vi "S4GUI.vi"(7 "Tab ObsEng":enum32{"Obs", "CCD modes", "Guider", "Eng"}(tab)) -> ()   [LabVIEW 2018] (continued)
        n1953 = event-data() -> ()  [unwired: 1 in, 6 out]
        n1954 = disable-structure shown="Disabled" {
          disable-tunnel: w3779 -> [w3791 _]
          frame Disabled {
            # "como alterar o valor de um parametro em \"Parameter Input\""
            n1955 = Unbundle By Name(w3791) -> ("Parameters"=w3793:T5)
            n1956 = Bundle By Name(cluster=w3793, "Readout\nRate"=u8 1 ("Readout\nRate")) -> (w3790:T5)
            n1957 = Bundle By Name(cluster=w3791, "Parameters"=w3790) -> (w3789:T8)
            n1958 = local write "Input Cluster"(w3789) -> ()
          }
          frame Enabled {
          }
        }
        n1959 = property on="Scrollbar" class="Scroll (strict)"() -> ("DocMax"=w3783:dbl)  [unwired: 2 in, 2 out]
        n1960 = Unbundle(w3781) -> ("Parameters"=w3786:refnum<vi>, "Current Configuration"=w3785:refnum<vi>)
        n1961 = Subtract(x=w3783, y="Scrollbar") -> (x-y=w3787:dbl)
        n1962 = Subtract(x=w3787, y=200.0 ("BarOffset")) -> (x-y=w3784:dbl)
        n1963 = property on="Property Node" class="Clust (strict)"(reference=w3786, "Top"=w3784) -> ()  [unwired: 1 in, 2 out]
        n1964 = property on="Property Node" class="Clust (strict)"(reference=w3785, "Top"=w3784) -> ()  [unwired: 1 in, 2 out]
      }
      event "Select Positions": Value Change {
        # "Garantir que, quando em POLARIMETRIA, pelo menos WP1 esteja selecionado."
        n1965 = event-data() -> ()  [unwired: 1 in, 6 out]
        n1966 = call "Read Instrument.lvclass.vi"("error in (no error)"=w3879, "S4ACS_GUI in"=w3878) -> ("error out"=w3887:errorcluster, "Instrument.lvclass"=w3886:refnum<class "Instrument.lvclass">, "S4ACS_GUI out"=w3881:refnum<class "S4GUI.lvclass">)  [unwired: 7 in]
        n1967 = call "Read WPROT.vi"("error in (no error)"=w3887, "Instrument in"=w3886) -> ("error out"=w3880:errorcluster, "Opt_Selector.lvclass"=w3883:refnum<class "Opt_Selector.lvclass">, "Instrument out"=w3882:refnum<class "Instrument.lvclass">)  [unwired: 7 in]
        n1968 = case shown="4" "Select Positions" {
          tunnel: w3880 -> [w3924 w3937 w3950 w3963 w3976 w3985]
          tunnel: [w3922 w3935 w3948 w3959 w3974 w3983] -> w3798
          tunnel: [w3920 w3933 w3946 w3960 w3972 w3984] -> w3796
          tunnel: w3883 -> [w3925 w3938 w3951 w3964 w3977 w3986]
          tunnel: [16 8 4 8 0 0] -> w3877
          tunnel: [0.0 ("Scale.Range:Minimum") 0.0 ("Scale.Range:Minimum") 0.0 ("Scale.Range:Minimum") 0.0 ("Scale.Range:Minimum") 0.0 ("Scale.Range:Minimum") 0.0 ("Scale.Range:Minimum")] -> w3876
          tunnel: [w3917 w3930 w3943 w3956 w3969 w3982] -> w3797
          frame 0, Default {
            w3917 = u16 65535 ("sequencia")
            w3926 = TRUE ("P0")
            w3927 = TRUE ("P0")
            w3928 = TRUE ("P0")
            w3929 = TRUE ("P0")
            # "1111 1111 1111 1111 = 65.535"
            n1969 = local write "P0"(w3929) -> ()
            n1970 = local write "P1"(w3929) -> ()
            n1971 = local write "P2"(w3929) -> ()
            n1972 = local write "P3"(w3929) -> ()
            n1973 = local write "P4"(w3927) -> ()
            n1974 = local write "P5"(w3927) -> ()
            n1975 = local write "P6"(w3927) -> ()
            n1976 = local write "P7"(w3927) -> ()
            n1977 = call-dynamic "Write sequencia.vi"("error in (no error)"=w3924, "sequencia"=w3917, "Opt_Selector in"=w3925) -> ("error out"=w3921:errorcluster, "Opt_Selector out"=w3923:refnum<class "Opt_Selector.lvclass">)  [unwired: 7 in]
            n1978 = call-dynamic "Write sequencia_ant.vi"("error in (no error)"=w3921, "sequencia_ant"=w3917, "Opt_Selector in"=w3923) -> ("error out"=w3920:errorcluster, "Opt_Selector out"=w3922:refnum<class "Opt_Selector.lvclass">)  [unwired: 7 in]
            n1979 = local write "P8"(w3928) -> ()
            n1980 = local write "P9"(w3928) -> ()
            n1981 = local write "P10"(w3928) -> ()
            n1982 = local write "P11"(w3928) -> ()
            n1983 = local write "P12"(w3926) -> ()
            n1984 = local write "P13"(w3926) -> ()
            n1985 = local write "P14"(w3926) -> ()
            n1986 = local write "P15"(w3926) -> ()
          }
          frame 1 {
            w3930 = u16 255 ("sequencia")
            w3939 = FALSE ("P0")
            w3940 = TRUE ("P0")
            w3941 = FALSE ("P0")
            w3942 = TRUE ("P0")
            # "0000 0000 1111 1111 = 255"
            n1987 = local write "P0"(w3942) -> ()
            n1988 = local write "P1"(w3942) -> ()
            n1989 = local write "P2"(w3942) -> ()
            n1990 = local write "P3"(w3942) -> ()
            n1991 = local write "P4"(w3940) -> ()
            n1992 = local write "P5"(w3940) -> ()
            n1993 = local write "P6"(w3940) -> ()
            n1994 = local write "P7"(w3940) -> ()
            n1995 = call-dynamic "Write sequencia.vi"("error in (no error)"=w3937, "sequencia"=w3930, "Opt_Selector in"=w3938) -> ("error out"=w3934:errorcluster, "Opt_Selector out"=w3936:refnum<class "Opt_Selector.lvclass">)  [unwired: 7 in]
            n1996 = local write "P8"(w3941) -> ()
            n1997 = local write "P9"(w3941) -> ()
            n1998 = local write "P10"(w3941) -> ()
            n1999 = local write "P11"(w3941) -> ()
            n2000 = local write "P12"(w3939) -> ()
            n2001 = local write "P13"(w3939) -> ()
            n2002 = local write "P14"(w3939) -> ()
            n2003 = local write "P15"(w3939) -> ()
            n2004 = call-dynamic "Write sequencia_ant.vi"("error in (no error)"=w3934, "sequencia_ant"=w3930, "Opt_Selector in"=w3936) -> ("error out"=w3933:errorcluster, "Opt_Selector out"=w3935:refnum<class "Opt_Selector.lvclass">)  [unwired: 7 in]
          }
          frame 2 {
            w3943 = u16 15 ("sequencia")
            w3952 = FALSE ("P0")
            w3953 = FALSE ("P0")
            w3954 = FALSE ("P0")
            w3955 = TRUE ("P0")
            # "0000 0000 0000 1111 = 15"
            n2005 = local write "P0"(w3955) -> ()
            n2006 = local write "P1"(w3955) -> ()
            n2007 = local write "P2"(w3955) -> ()
            n2008 = local write "P3"(w3955) -> ()
            n2009 = local write "P4"(w3953) -> ()
            n2010 = local write "P5"(w3953) -> ()
            n2011 = local write "P6"(w3953) -> ()
            n2012 = local write "P7"(w3953) -> ()
            n2013 = call-dynamic "Write sequencia.vi"("error in (no error)"=w3950, "sequencia"=w3943, "Opt_Selector in"=w3951) -> ("error out"=w3947:errorcluster, "Opt_Selector out"=w3949:refnum<class "Opt_Selector.lvclass">)  [unwired: 7 in]
            n2014 = call-dynamic "Write sequencia_ant.vi"("error in (no error)"=w3947, "sequencia_ant"=w3943, "Opt_Selector in"=w3949) -> ("error out"=w3946:errorcluster, "Opt_Selector out"=w3948:refnum<class "Opt_Selector.lvclass">)  [unwired: 7 in]
            n2015 = local write "P8"(w3954) -> ()
            n2016 = local write "P9"(w3954) -> ()
            n2017 = local write "P10"(w3954) -> ()
            n2018 = local write "P11"(w3954) -> ()
            n2019 = local write "P12"(w3952) -> ()
            n2020 = local write "P13"(w3952) -> ()
            n2021 = local write "P14"(w3952) -> ()
            n2022 = local write "P15"(w3952) -> ()
          }
          frame 3 {
            w3956 = u16 3855 ("sequencia")
            w3965 = FALSE ("P0")
            w3966 = FALSE ("P0")
            w3967 = TRUE ("P0")
            w3968 = TRUE ("P0")
            # "0000 1111 0000 1111 = 3855"
            n2023 = local write "P0"(w3968) -> ()
            n2024 = local write "P1"(w3968) -> ()
            n2025 = local write "P2"(w3968) -> ()
            n2026 = local write "P3"(w3968) -> ()
            n2027 = local write "P4"(w3966) -> ()
            n2028 = local write "P5"(w3966) -> ()
            n2029 = local write "P6"(w3966) -> ()
            n2030 = local write "P7"(w3966) -> ()
            n2031 = call-dynamic "Write sequencia.vi"("error in (no error)"=w3963, "sequencia"=w3956, "Opt_Selector in"=w3964) -> ("error out"=w3961:errorcluster, "Opt_Selector out"=w3962:refnum<class "Opt_Selector.lvclass">)  [unwired: 7 in]
            n2032 = local write "P8"(w3967) -> ()
            n2033 = local write "P9"(w3967) -> ()
            n2034 = local write "P10"(w3967) -> ()
            n2035 = local write "P11"(w3967) -> ()
            n2036 = local write "P12"(w3965) -> ()
            n2037 = local write "P13"(w3965) -> ()
            n2038 = local write "P14"(w3965) -> ()
            n2039 = local write "P15"(w3965) -> ()
            n2040 = call-dynamic "Write sequencia_ant.vi"("error in (no error)"=w3961, "sequencia_ant"=w3956, "Opt_Selector in"=w3962) -> ("error out"=w3960:errorcluster, "Opt_Selector out"=w3959:refnum<class "Opt_Selector.lvclass">)  [unwired: 7 in]
          }
          frame 4 {
            w3969 = u16 0 ("sequencia")
            w3978 = FALSE ("P0")
            w3979 = FALSE ("P0")
            w3980 = FALSE ("P0")
            w3981 = FALSE ("P0")
            n2041 = local write "P0"(w3981) -> ()
            n2042 = local write "P1"(w3981) -> ()
            n2043 = local write "P2"(w3981) -> ()
            n2044 = local write "P3"(w3981) -> ()
            n2045 = local write "P4"(w3979) -> ()
            n2046 = local write "P5"(w3979) -> ()
            n2047 = local write "P6"(w3979) -> ()
            n2048 = local write "P7"(w3979) -> ()
            n2049 = call-dynamic "Write sequencia.vi"("error in (no error)"=w3976, "sequencia"=w3969, "Opt_Selector in"=w3977) -> ("error out"=w3973:errorcluster, "Opt_Selector out"=w3975:refnum<class "Opt_Selector.lvclass">)  [unwired: 7 in]
            n2050 = call-dynamic "Write sequencia_ant.vi"("error in (no error)"=w3973, "sequencia_ant"=w3969, "Opt_Selector in"=w3975) -> ("error out"=w3972:errorcluster, "Opt_Selector out"=w3974:refnum<class "Opt_Selector.lvclass">)  [unwired: 7 in]
            n2051 = local write "P8"(w3980) -> ()
            n2052 = local write "P9"(w3980) -> ()
            n2053 = local write "P10"(w3980) -> ()
            n2054 = local write "P11"(w3980) -> ()
            n2055 = local write "P12"(w3978) -> ()
            n2056 = local write "P13"(w3978) -> ()
            n2057 = local write "P14"(w3978) -> ()
            n2058 = local write "P15"(w3978) -> ()
          }
          frame 5 {
            n2059 = call-dynamic "Read sequencia_ant.vi"("error in (no error)"=w3985, "Opt_Selector in"=w3986) -> ("error out"=w3984:errorcluster, "sequencia_ant"=w3982:u16, "Opt_Selector out"=w3983:refnum<class "Opt_Selector.lvclass">)  [unwired: 7 in]
          }
        }
        n2060 = call-dynamic "Write prev_sequencia.vi"("error in (no error)"=w3796, "prev_sequencia"=w3797, "Opt_Selector in"=w3798) -> ("error out"=w3795:errorcluster, "Opt_Selector out"=w3794:refnum<class "Opt_Selector.lvclass">)  [unwired: 7 in]
        n2061 = call "Write WPROT.vi"("error in (no error)"=w3795, "Opt_Selector.lvclass"=w3794, "Instrument in"=w3882) -> ("error out"=w3884:errorcluster, "Instrument out"=w3885:refnum<class "Instrument.lvclass">)  [unwired: 7 in]
        n2062 = property on="#Pol. Seq. Done" class="Slide (strict)"(error in=w3795, "Scale.Maximum"=w3877, "Scale.Minimum"=w3876) -> ()  [unwired: 1 in, 2 out]
        n2063 = call "Write Instrument.lvclass.vi"("error in (no error)"=w3884, "Instrument.lvclass"=w3885, "S4ACS_GUI in"=w3881) -> ("error out"=w3866:errorcluster, "S4ACS_GUI out"=w3867:refnum<class "S4GUI.lvclass">)  [unwired: 7 in]
        n2064 = call "Read Instrument.lvclass.vi"("error in (no error)"=w3866, "S4ACS_GUI in"=w3867) -> ("error out"=w3871:errorcluster, "Instrument.lvclass"=w3872:refnum<class "Instrument.lvclass">, "S4ACS_GUI out"=w3875:refnum<class "S4GUI.lvclass">)  [unwired: 7 in]
        n2065 = call "Read ASEL.vi"("error in (no error)"=w3871, "Instrument in"=w3872) -> ("error out"=w3863:errorcluster, "Opt_Selector.lvclass"=w3865:refnum<class "Opt_Selector.lvclass">, "Instrument out"=w3868:refnum<class "Instrument.lvclass">)  [unwired: 7 in]
        n2066 = call "Read name_pos.vi"("error in (no error)"=w3863, "Optics in"=w3865) -> ("error out"=w3862:errorcluster, "name_pos"=w3861:string, "Optics out"=w3864:refnum<class "Opt_Selector.lvclass">)  [unwired: 7 in]
        n2067 = call "Write ASEL.vi"("error in (no error)"=w3862, "Opt_Selector.lvclass"=w3864, "Instrument in"=w3868) -> ("error out"=w3869:errorcluster, "Instrument out"=w3873:refnum<class "Instrument.lvclass">)  [unwired: 7 in]
        n2068 = case shown="\"ON\"" w3861 {
          tunnel: w3869 -> [w3890 w3901]
          tunnel: [w3890 w3897] -> w3870
          tunnel: w3873 -> [w3889 w3902]
          tunnel: [w3889 w3898] -> w3874
          frame Default {
          }
          frame "ON" {
            n2069 = call "Read WPROT.vi"("error in (no error)"=w3901, "Instrument in"=w3902) -> ("error out"=w3893:errorcluster, "Opt_Selector.lvclass"=w3900:refnum<class "Opt_Selector.lvclass">, "Instrument out"=w3899:refnum<class "Instrument.lvclass">)  [unwired: 7 in]
            n2070 = call-dynamic "Read sequencia.vi"("error in (no error)"=w3893, "Opt_Selector in"=w3900) -> ("error out"=w3892:errorcluster, "sequencia"=w3896:u16, "Opt_Selector out"=w3895:refnum<class "Opt_Selector.lvclass">)  [unwired: 7 in]
            n2071 = case shown="0" w3896 {
              tunnel: w3895 -> [w3904 w3916]
              tunnel: [w3904 w3908] -> w3894
              tunnel: w3892 -> [w3903 w3915]
              tunnel: [w3903 w3906] -> w3891
              frame Default {
              }
              frame 0 {
                n2072 = call-dynamic "Write sequencia.vi"("error in (no error)"=w3915, "sequencia"=u16 1, "Opt_Selector in"=w3916) -> ("error out"=w3912:errorcluster, "Opt_Selector out"=w3913:refnum<class "Opt_Selector.lvclass">)  [unwired: 7 in]
                n2073 = local write "P0"(TRUE ("P0")) -> ()
                n2074 = call-dynamic "Write sequencia_ant.vi"("error in (no error)"=w3912, "sequencia_ant"=u16 1, "Opt_Selector in"=w3913) -> ("error out"=w3907:errorcluster, "Opt_Selector out"=w3909:refnum<class "Opt_Selector.lvclass">)  [unwired: 7 in]
                n2075 = call-dynamic "Write prev_sequencia.vi"("error in (no error)"=w3907, "prev_sequencia"=u16 1, "Opt_Selector in"=w3909) -> ("error out"=w3906:errorcluster, "Opt_Selector out"=w3908:refnum<class "Opt_Selector.lvclass">)  [unwired: 7 in]
              }
            }
            n2076 = call "Write WPROT.vi"("error in (no error)"=w3891, "Opt_Selector.lvclass"=w3894, "Instrument in"=w3899) -> ("error out"=w3897:errorcluster, "Instrument out"=w3898:refnum<class "Instrument.lvclass">)  [unwired: 7 in]
          }
        }
        n2077 = call "Write Instrument.lvclass.vi"("error in (no error)"=w3870, "Instrument.lvclass"=w3874, "S4ACS_GUI in"=w3875) -> ("error out"=w3799:errorcluster, "S4ACS_GUI out"=w3800:refnum<class "S4GUI.lvclass">)  [unwired: 7 in]
        n2078 = call-dynamic "Read AcquisitionA.vi"("error in (no error)"=w3799, "S4ACS_GUI in"=w3800) -> ("error out"=w3858:errorcluster, "Acquisition.lvclass"=w3860:refnum<class "Acquisition.lvclass">, "S4ACS_GUI out"=w3857:refnum<class "S4GUI.lvclass">)  [unwired: 7 in]
        n2079 = call-dynamic "Read Channel.vi"("error in (no error)"=w3858, "Acquisition in"=w3860) -> ("error out"=w3854:errorcluster, "Channel.lvclass"=w3855:refnum<class "Channel.lvclass">, "Acquisition out"=w3859:refnum<class "Acquisition.lvclass">)  [unwired: 7 in]
        n2080 = call-dynamic "Write sequencias.vi"("error in (no error)"=w3854, "sequencias"=w3797, "Channel in"=w3855) -> ("error out"=w3851:errorcluster, "Channel out"=w3853:refnum<class "Channel.lvclass">)  [unwired: 7 in]
        n2081 = call-dynamic "Write prev sequencias.vi"("error in (no error)"=w3851, "prev sequencias"=w3797, "Channel in"=w3853) -> ("error out"=w3850:errorcluster, "Channel out"=w3852:refnum<class "Channel.lvclass">)  [unwired: 7 in]
        n2082 = call-dynamic "Write Channel.vi"("error in (no error)"=w3850, "Channel.lvclass"=w3852, "Acquisition in"=w3859) -> ("error out"=w3849:errorcluster, "Acquisition out"=w3856:refnum<class "Acquisition.lvclass">)  [unwired: 7 in]
        n2083 = call-dynamic "Write AcquisitionA.vi"("error in (no error)"=w3849, "Acquisition.lvclass"=w3856, "S4ACS_GUI in"=w3857) -> ("error out"=w3807:errorcluster, "S4ACS_GUI out"=w3808:refnum<class "S4GUI.lvclass">)  [unwired: 7 in]
        n2084 = call "Read AcquisitionB.vi"("error in (no error)"=w3807, "S4ACS_GUI in"=w3808) -> ("error out"=w3834:errorcluster, "Acquisition.lvclass"=w3836:refnum<class "Acquisition.lvclass">, "S4ACS_GUI out"=w3833:refnum<class "S4GUI.lvclass">)  [unwired: 7 in]
        n2085 = call-dynamic "Read Channel.vi"("error in (no error)"=w3834, "Acquisition in"=w3836) -> ("error out"=w3830:errorcluster, "Channel.lvclass"=w3831:refnum<class "Channel.lvclass">, "Acquisition out"=w3835:refnum<class "Acquisition.lvclass">)  [unwired: 7 in]
        n2086 = call-dynamic "Write sequencias.vi"("error in (no error)"=w3830, "sequencias"=w3797, "Channel in"=w3831) -> ("error out"=w3827:errorcluster, "Channel out"=w3829:refnum<class "Channel.lvclass">)  [unwired: 7 in]
        n2087 = call-dynamic "Write prev sequencias.vi"("error in (no error)"=w3827, "prev sequencias"=w3797, "Channel in"=w3829) -> ("error out"=w3826:errorcluster, "Channel out"=w3828:refnum<class "Channel.lvclass">)  [unwired: 7 in]
        n2088 = call-dynamic "Write Channel.vi"("error in (no error)"=w3826, "Channel.lvclass"=w3828, "Acquisition in"=w3835) -> ("error out"=w3825:errorcluster, "Acquisition out"=w3832:refnum<class "Acquisition.lvclass">)  [unwired: 7 in]
        n2089 = call "Write AcquisitionB.vi"("error in (no error)"=w3825, "Acquisition.lvclass"=w3832, "S4ACS_GUI in"=w3833) -> ("error out"=w3809:errorcluster, "S4ACS_GUI out"=w3810:refnum<class "S4GUI.lvclass">)  [unwired: 7 in]
        n2090 = call-dynamic "Read AcquisitionC.vi"("error in (no error)"=w3809, "S4ACS_GUI in"=w3810) -> ("error out"=w3822:errorcluster, "Acquisition.lvclass"=w3824:refnum<class "Acquisition.lvclass">, "S4ACS_GUI out"=w3821:refnum<class "S4GUI.lvclass">)  [unwired: 7 in]
        n2091 = call-dynamic "Read Channel.vi"("error in (no error)"=w3822, "Acquisition in"=w3824) -> ("error out"=w3818:errorcluster, "Channel.lvclass"=w3819:refnum<class "Channel.lvclass">, "Acquisition out"=w3823:refnum<class "Acquisition.lvclass">)  [unwired: 7 in]
        n2092 = call-dynamic "Write sequencias.vi"("error in (no error)"=w3818, "sequencias"=w3797, "Channel in"=w3819) -> ("error out"=w3815:errorcluster, "Channel out"=w3817:refnum<class "Channel.lvclass">)  [unwired: 7 in]
        n2093 = call-dynamic "Write prev sequencias.vi"("error in (no error)"=w3815, "prev sequencias"=w3797, "Channel in"=w3817) -> ("error out"=w3814:errorcluster, "Channel out"=w3816:refnum<class "Channel.lvclass">)  [unwired: 7 in]
        n2094 = call-dynamic "Write Channel.vi"("error in (no error)"=w3814, "Channel.lvclass"=w3816, "Acquisition in"=w3823) -> ("error out"=w3813:errorcluster, "Acquisition out"=w3820:refnum<class "Acquisition.lvclass">)  [unwired: 7 in]
        n2095 = call-dynamic "Write AcquisitionC.vi"("error in (no error)"=w3813, "Acquisition.lvclass"=w3820, "S4ACS_GUI in"=w3821) -> ("error out"=w3805:errorcluster, "S4ACS_GUI out"=w3806:refnum<class "S4GUI.lvclass">)  [unwired: 7 in]
        n2096 = call-dynamic "Read AcquisitionD.vi"("error in (no error)"=w3805, "S4ACS_GUI in"=w3806) -> ("error out"=w3846:errorcluster, "Acquisition.lvclass"=w3848:refnum<class "Acquisition.lvclass">, "S4ACS_GUI out"=w3845:refnum<class "S4GUI.lvclass">)  [unwired: 7 in]
        n2097 = call-dynamic "Read Channel.vi"("error in (no error)"=w3846, "Acquisition in"=w3848) -> ("error out"=w3842:errorcluster, "Channel.lvclass"=w3843:refnum<class "Channel.lvclass">, "Acquisition out"=w3847:refnum<class "Acquisition.lvclass">)  [unwired: 7 in]
        n2098 = call-dynamic "Write sequencias.vi"("error in (no error)"=w3842, "sequencias"=w3797, "Channel in"=w3843) -> ("error out"=w3839:errorcluster, "Channel out"=w3841:refnum<class "Channel.lvclass">)  [unwired: 7 in]
        n2099 = call-dynamic "Write prev sequencias.vi"("error in (no error)"=w3839, "prev sequencias"=w3797, "Channel in"=w3841) -> ("error out"=w3838:errorcluster, "Channel out"=w3840:refnum<class "Channel.lvclass">)  [unwired: 7 in]
        n2100 = call-dynamic "Write Channel.vi"("error in (no error)"=w3838, "Channel.lvclass"=w3840, "Acquisition in"=w3847) -> ("error out"=w3837:errorcluster, "Acquisition out"=w3844:refnum<class "Acquisition.lvclass">)  [unwired: 7 in]
        n2101 = call-dynamic "Write AcquisitionD.vi"("error in (no error)"=w3837, "Acquisition.lvclass"=w3844, "S4ACS_GUI in"=w3845) -> ("error out"=w3803:errorcluster, "S4ACS_GUI out"=w3804:refnum<class "S4GUI.lvclass">)  [unwired: 7 in]
        n2102 = call-dynamic "Write sequencias.vi"("error in (no error)"=w3803, "sequencias"=w3797, "S4GUI in"=w3804) -> ("error out"=w3812:errorcluster, "S4GUI out"=w3811:refnum<class "S4GUI.lvclass">)  [unwired: 7 in]
        n2103 = call-dynamic "Write prev sequencias.vi"("error in (no error)"=w3812, "prev sequencias"=w3797, "S4GUI in"=w3811) -> ("error out"=w3801:errorcluster, "S4GUI out"=w3802:refnum<class "S4GUI.lvclass">)  [unwired: 7 in]
      }
      event "P0", "P1", "P2", "P3", "P4", "P5", "P6", "P7", "P8", "P9", "P10", "P11", "P12", "P13", "P14", "P15": Value Change {
        w4104 = u16 5 items=["All 16 positions", "First 8 positions", "First 4 positions", "0-3 + 8-11", "Clear", "Customized"] ("Select Positions")
        # "Garantir que, quando em POLARIMETRIA, pelo menos WP1 esteja selecionado."
        # "Salva tambem em \nSequencia_ant para\no caso de repeticao.\n\nE salva em PrevSeq para\nrecuperar a ultima sequencia\ndepois de passar pela aba TEST."
        n2104 = event-data() -> ()  [unwired: 1 in, 6 out]
        n2105 = local write "Select Positions"(w4104) -> ()
        n2106 = call "Read Instrument.lvclass.vi"("error in (no error)"=w4086, "S4ACS_GUI in"=w4087) -> ("error out"=w4081:errorcluster, "Instrument.lvclass"=w4084:refnum<class "Instrument.lvclass">, "S4ACS_GUI out"=w4085:refnum<class "S4GUI.lvclass">)  [unwired: 7 in]
        n2107 = Build Array("P0", "P1", "P2", "P3", "P4", "P5", "P6", "P7", "P8", "P9", "P10", "P11", "P12", "P13", "P14", "P15") -> (w4075:bool[])
        n2108 = call "Read WPROT.vi"("error in (no error)"=w4081, "Instrument in"=w4084) -> ("error out"=w4080:errorcluster, "Opt_Selector.lvclass"=w4082:refnum<class "Opt_Selector.lvclass">, "Instrument out"=w4083:refnum<class "Instrument.lvclass">)  [unwired: 7 in]
        n2109 = Boolean Array To Number(Boolean array=w4075) -> (number=w4088:u32)
        n2110 = To Unsigned Word Integer(number=w4088) -> (unsigned 16bit integer=w3989:u16)
        n2111 = call-dynamic "Write sequencia.vi"("error in (no error)"=w4080, "sequencia"=w3989, "Opt_Selector in"=w4082) -> ("error out"=w4076:errorcluster, "Opt_Selector out"=w4077:refnum<class "Opt_Selector.lvclass">)  [unwired: 7 in]
        n2112 = call-dynamic "Write sequencia_ant.vi"("error in (no error)"=w4076, "sequencia_ant"=w3989, "Opt_Selector in"=w4077) -> ("error out"=w3992:errorcluster, "Opt_Selector out"=w3993:refnum<class "Opt_Selector.lvclass">)  [unwired: 7 in]
        n2113 = call-dynamic "Write prev_sequencia.vi"("error in (no error)"=w3992, "prev_sequencia"=w3989, "Opt_Selector in"=w3993) -> ("error out"=w3991:errorcluster, "Opt_Selector out"=w3990:refnum<class "Opt_Selector.lvclass">)  [unwired: 7 in]
        n2114 = call "Write WPROT.vi"("error in (no error)"=w3991, "Opt_Selector.lvclass"=w3990, "Instrument in"=w4083) -> ("error out"=w4079:errorcluster, "Instrument out"=w4078:refnum<class "Instrument.lvclass">)  [unwired: 7 in]
        n2115 = call "Write Instrument.lvclass.vi"("error in (no error)"=w4079, "Instrument.lvclass"=w4078, "S4ACS_GUI in"=w4085) -> ("error out"=w4056:errorcluster, "S4ACS_GUI out"=w4057:refnum<class "S4GUI.lvclass">)  [unwired: 7 in]
        n2116 = call "Read Instrument.lvclass.vi"("error in (no error)"=w4056, "S4ACS_GUI in"=w4057) -> ("error out"=w4062:errorcluster, "Instrument.lvclass"=w4061:refnum<class "Instrument.lvclass">, "S4ACS_GUI out"=w4058:refnum<class "S4GUI.lvclass">)  [unwired: 7 in]
        n2117 = call "Read ASEL.vi"("error in (no error)"=w4062, "Instrument in"=w4061) -> ("error out"=w4068:errorcluster, "Opt_Selector.lvclass"=w4066:refnum<class "Opt_Selector.lvclass">, "Instrument out"=w4065:refnum<class "Instrument.lvclass">)  [unwired: 7 in]
        n2118 = call "Read name_pos.vi"("error in (no error)"=w4068, "Optics in"=w4066) -> ("error out"=w4069:errorcluster, "name_pos"=w4070:string, "Optics out"=w4067:refnum<class "Opt_Selector.lvclass">)  [unwired: 7 in]
        n2119 = call "Write ASEL.vi"("error in (no error)"=w4069, "Opt_Selector.lvclass"=w4067, "Instrument in"=w4065) -> ("error out"=w4064:errorcluster, "Instrument out"=w4060:refnum<class "Instrument.lvclass">)  [unwired: 7 in]
        n2120 = case shown="\"ON\"" w4070 {
          tunnel: w4064 -> [w4106 w4117]
          tunnel: [w4106 w4113] -> w4063
          tunnel: w4060 -> [w4105 w4118]
          tunnel: [w4105 w4114] -> w4059
          frame Default {
          }
          frame "ON" {
            n2121 = call "Read WPROT.vi"("error in (no error)"=w4117, "Instrument in"=w4118) -> ("error out"=w4109:errorcluster, "Opt_Selector.lvclass"=w4116:refnum<class "Opt_Selector.lvclass">, "Instrument out"=w4115:refnum<class "Instrument.lvclass">)  [unwired: 7 in]
            n2122 = call-dynamic "Read sequencia.vi"("error in (no error)"=w4109, "Opt_Selector in"=w4116) -> ("error out"=w4108:errorcluster, "sequencia"=w4112:u16, "Opt_Selector out"=w4111:refnum<class "Opt_Selector.lvclass">)  [unwired: 7 in]
            n2123 = case shown="0" w4112 {
              tunnel: w4111 -> [w4120 w4132]
              tunnel: [w4120 w4123] -> w4110
              tunnel: w4108 -> [w4119 w4131]
              tunnel: [w4119 w4122] -> w4107
              frame Default {
              }
              frame 0 {
                n2124 = call-dynamic "Write sequencia.vi"("error in (no error)"=w4131, "sequencia"=u16 1, "Opt_Selector in"=w4132) -> ("error out"=w4128:errorcluster, "Opt_Selector out"=w4129:refnum<class "Opt_Selector.lvclass">)  [unwired: 7 in]
                n2125 = local write "P0"(TRUE ("P0")) -> ()
                n2126 = call-dynamic "Write sequencia_ant.vi"("error in (no error)"=w4128, "sequencia_ant"=u16 1, "Opt_Selector in"=w4129) -> ("error out"=w4124:errorcluster, "Opt_Selector out"=w4125:refnum<class "Opt_Selector.lvclass">)  [unwired: 7 in]
                n2127 = call-dynamic "Write prev_sequencia.vi"("error in (no error)"=w4124, "prev_sequencia"=u16 1, "Opt_Selector in"=w4125) -> ("error out"=w4122:errorcluster, "Opt_Selector out"=w4123:refnum<class "Opt_Selector.lvclass">)  [unwired: 7 in]
              }
            }
            n2128 = call "Write WPROT.vi"("error in (no error)"=w4107, "Opt_Selector.lvclass"=w4110, "Instrument in"=w4115) -> ("error out"=w4113:errorcluster, "Instrument out"=w4114:refnum<class "Instrument.lvclass">)  [unwired: 7 in]
          }
        }
        n2129 = for {
          tunnel: w4075 -> [w4136] mode=indexing
          shift-right: [w4135] -> w4073
          shift-left: 0 -> [w4133]
          # "calcula qtd de 1s"
          n2130 = Increment(x=w4133) -> (x+1=w4134:i32)
          n2131 = Select(t=w4134, s=w4136, f=w4133) -> (s? t:f=w4135:i32)
        }
        n2132 = property on="#Pol. Seq. Done" class="Slide (strict)"("Scale.Maximum"=w4073, "Scale.Minimum"=0.0 ("Scale.Range:Minimum")) -> ()  [unwired: 2 in, 2 out]
        n2133 = call "Write Instrument.lvclass.vi"("error in (no error)"=w4063, "Instrument.lvclass"=w4059, "S4ACS_GUI in"=w4058) -> ("error out"=w4000:errorcluster, "S4ACS_GUI out"=w4001:refnum<class "S4GUI.lvclass">)  [unwired: 7 in]
        n2134 = call-dynamic "Read AcquisitionA.vi"("error in (no error)"=w4000, "S4ACS_GUI in"=w4001) -> ("error out"=w4053:errorcluster, "Acquisition.lvclass"=w4055:refnum<class "Acquisition.lvclass">, "S4ACS_GUI out"=w4052:refnum<class "S4GUI.lvclass">)  [unwired: 7 in]
        n2135 = call-dynamic "Read Channel.vi"("error in (no error)"=w4053, "Acquisition in"=w4055) -> ("error out"=w4049:errorcluster, "Channel.lvclass"=w4050:refnum<class "Channel.lvclass">, "Acquisition out"=w4054:refnum<class "Acquisition.lvclass">)  [unwired: 7 in]
        n2136 = call-dynamic "Write sequencias.vi"("error in (no error)"=w4049, "sequencias"=w3989, "Channel in"=w4050) -> ("error out"=w4046:errorcluster, "Channel out"=w4048:refnum<class "Channel.lvclass">)  [unwired: 7 in]
        n2137 = call-dynamic "Write prev sequencias.vi"("error in (no error)"=w4046, "prev sequencias"=w3989, "Channel in"=w4048) -> ("error out"=w4045:errorcluster, "Channel out"=w4047:refnum<class "Channel.lvclass">)  [unwired: 7 in]
        n2138 = call-dynamic "Write Channel.vi"("error in (no error)"=w4045, "Channel.lvclass"=w4047, "Acquisition in"=w4054) -> ("error out"=w4044:errorcluster, "Acquisition out"=w4051:refnum<class "Acquisition.lvclass">)  [unwired: 7 in]
        n2139 = call-dynamic "Write AcquisitionA.vi"("error in (no error)"=w4044, "Acquisition.lvclass"=w4051, "S4ACS_GUI in"=w4052) -> ("error out"=w3998:errorcluster, "S4ACS_GUI out"=w3999:refnum<class "S4GUI.lvclass">)  [unwired: 7 in]
        n2140 = call "Read AcquisitionB.vi"("error in (no error)"=w3998, "S4ACS_GUI in"=w3999) -> ("error out"=w4029:errorcluster, "Acquisition.lvclass"=w4031:refnum<class "Acquisition.lvclass">, "S4ACS_GUI out"=w4028:refnum<class "S4GUI.lvclass">)  [unwired: 7 in]
        n2141 = call-dynamic "Read Channel.vi"("error in (no error)"=w4029, "Acquisition in"=w4031) -> ("error out"=w4025:errorcluster, "Channel.lvclass"=w4026:refnum<class "Channel.lvclass">, "Acquisition out"=w4030:refnum<class "Acquisition.lvclass">)  [unwired: 7 in]
        n2142 = call-dynamic "Write sequencias.vi"("error in (no error)"=w4025, "sequencias"=w3989, "Channel in"=w4026) -> ("error out"=w4022:errorcluster, "Channel out"=w4024:refnum<class "Channel.lvclass">)  [unwired: 7 in]
        n2143 = call-dynamic "Write prev sequencias.vi"("error in (no error)"=w4022, "prev sequencias"=w3989, "Channel in"=w4024) -> ("error out"=w4021:errorcluster, "Channel out"=w4023:refnum<class "Channel.lvclass">)  [unwired: 7 in]
        n2144 = call-dynamic "Write Channel.vi"("error in (no error)"=w4021, "Channel.lvclass"=w4023, "Acquisition in"=w4030) -> ("error out"=w4020:errorcluster, "Acquisition out"=w4027:refnum<class "Acquisition.lvclass">)  [unwired: 7 in]
        n2145 = call "Write AcquisitionB.vi"("error in (no error)"=w4020, "Acquisition.lvclass"=w4027, "S4ACS_GUI in"=w4028) -> ("error out"=w4002:errorcluster, "S4ACS_GUI out"=w4003:refnum<class "S4GUI.lvclass">)  [unwired: 7 in]
        n2146 = call-dynamic "Read AcquisitionC.vi"("error in (no error)"=w4002, "S4ACS_GUI in"=w4003) -> ("error out"=w4017:errorcluster, "Acquisition.lvclass"=w4019:refnum<class "Acquisition.lvclass">, "S4ACS_GUI out"=w4016:refnum<class "S4GUI.lvclass">)  [unwired: 7 in]
        n2147 = call-dynamic "Read Channel.vi"("error in (no error)"=w4017, "Acquisition in"=w4019) -> ("error out"=w4013:errorcluster, "Channel.lvclass"=w4014:refnum<class "Channel.lvclass">, "Acquisition out"=w4018:refnum<class "Acquisition.lvclass">)  [unwired: 7 in]
        n2148 = call-dynamic "Write sequencias.vi"("error in (no error)"=w4013, "sequencias"=w3989, "Channel in"=w4014) -> ("error out"=w4010:errorcluster, "Channel out"=w4012:refnum<class "Channel.lvclass">)  [unwired: 7 in]
        n2149 = call-dynamic "Write prev sequencias.vi"("error in (no error)"=w4010, "prev sequencias"=w3989, "Channel in"=w4012) -> ("error out"=w4009:errorcluster, "Channel out"=w4011:refnum<class "Channel.lvclass">)  [unwired: 7 in]
        n2150 = call-dynamic "Write Channel.vi"("error in (no error)"=w4009, "Channel.lvclass"=w4011, "Acquisition in"=w4018) -> ("error out"=w4008:errorcluster, "Acquisition out"=w4015:refnum<class "Acquisition.lvclass">)  [unwired: 7 in]
        n2151 = call-dynamic "Write AcquisitionC.vi"("error in (no error)"=w4008, "Acquisition.lvclass"=w4015, "S4ACS_GUI in"=w4016) -> ("error out"=w3996:errorcluster, "S4ACS_GUI out"=w3997:refnum<class "S4GUI.lvclass">)  [unwired: 7 in]
        n2152 = call-dynamic "Read AcquisitionD.vi"("error in (no error)"=w3996, "S4ACS_GUI in"=w3997) -> ("error out"=w4041:errorcluster, "Acquisition.lvclass"=w4043:refnum<class "Acquisition.lvclass">, "S4ACS_GUI out"=w4040:refnum<class "S4GUI.lvclass">)  [unwired: 7 in]
        n2153 = call-dynamic "Read Channel.vi"("error in (no error)"=w4041, "Acquisition in"=w4043) -> ("error out"=w4037:errorcluster, "Channel.lvclass"=w4038:refnum<class "Channel.lvclass">, "Acquisition out"=w4042:refnum<class "Acquisition.lvclass">)  [unwired: 7 in]
        n2154 = call-dynamic "Write sequencias.vi"("error in (no error)"=w4037, "sequencias"=w3989, "Channel in"=w4038) -> ("error out"=w4034:errorcluster, "Channel out"=w4036:refnum<class "Channel.lvclass">)  [unwired: 7 in]
        n2155 = call-dynamic "Write prev sequencias.vi"("error in (no error)"=w4034, "prev sequencias"=w3989, "Channel in"=w4036) -> ("error out"=w4033:errorcluster, "Channel out"=w4035:refnum<class "Channel.lvclass">)  [unwired: 7 in]
        n2156 = call-dynamic "Write Channel.vi"("error in (no error)"=w4033, "Channel.lvclass"=w4035, "Acquisition in"=w4042) -> ("error out"=w4032:errorcluster, "Acquisition out"=w4039:refnum<class "Acquisition.lvclass">)  [unwired: 7 in]
        n2157 = call-dynamic "Write AcquisitionD.vi"("error in (no error)"=w4032, "Acquisition.lvclass"=w4039, "S4ACS_GUI in"=w4040) -> ("error out"=w3994:errorcluster, "S4ACS_GUI out"=w3995:refnum<class "S4GUI.lvclass">)  [unwired: 7 in]
        n2158 = call-dynamic "Write sequencias.vi"("error in (no error)"=w3994, "sequencias"=w3989, "S4GUI in"=w3995) -> ("error out"=w4006:errorcluster, "S4GUI out"=w4005:refnum<class "S4GUI.lvclass">)  [unwired: 7 in]
        n2159 = call-dynamic "Write prev sequencias.vi"("error in (no error)"=w4006, "prev sequencias"=w3989, "S4GUI in"=w4005) -> ("error out"=w4007:errorcluster, "S4GUI out"=w4004:refnum<class "S4GUI.lvclass">)  [unwired: 7 in]
      }
      event "SSM": Value Change {
        # "F: fotom.\nT: polar."
        n2160 = event-data() -> ("NewVal"=w4144:u16)  [unwired: 1 in, 5 out]
        n2161 = call-dynamic "Read mode EXPOSE.vi"("error in (no error)"=w4150, "S4GUI in"=w4151) -> ("error out"=w4149:errorcluster, "mode EXPOSE"=w4145:bool, "S4GUI out"=w4146:refnum<class "S4GUI.lvclass">)  [unwired: 7 in]
        n2162 = call "Read Instrument.lvclass.vi"("error in (no error)"=w4149, "S4ACS_GUI in"=w4146) -> ("error out"=w4148:errorcluster, "Instrument.lvclass"=w4154:refnum<class "Instrument.lvclass">, "S4ACS_GUI out"=w4153:refnum<class "S4GUI.lvclass">)  [unwired: 7 in]
        n2163 = call-dynamic "Read mode.vi"("error in (no error)"=w4148, "Instrument in"=w4154) -> ("error out"=w4147:errorcluster, "mode"=w4152:bool)  [unwired: 7 in, 1 out]
        n2164 = case shown="1" w4144 {
          tunnel: [TRUE FALSE] -> w4157
          tunnel: w4147 -> [w4168 w4394]
          tunnel: w4153 -> [w4170 w4393]
          tunnel: [w4161 w4385] -> w4156
          tunnel: [w4160 w4384] -> w4155
          tunnel: w4152 -> [_ w4374]
          tunnel: w4145 -> [_ w4372]
          tunnel: ["SYNCHRONOUS" "ASYNCHRONOUS"] -> w4137
          frame 1 {
            # "Sync mode: Os canais sao configurados para Trigger externo, desde que o SyncBox esteja conectado."
            # "Sync by Cycle"
            n2165 = call-dynamic "Read Sync Box.lvclass.vi"("error in (no error)"=w4168, "SPARC4_AC in"=w4170) -> ("error out"=w4167:errorcluster, "Sync Box.lvclass"=w4171:refnum<class "Sync Box.lvclass">, "SPARC4_AC out"=w4169:refnum<class "S4GUI.lvclass">)  [unwired: 7 in]
            n2166 = call "Read connection.vi"("error in (no error)"=w4167, "Server in"=w4171) -> ("error out"=w4166:errorcluster, "connection"=w4165:bool)  [unwired: 7 in, 1 out]
            n2167 = case shown="False" w4165 {
              tunnel: [w4174 w4191] -> w4163
              tunnel: w4169 -> [w4174 w4181]
              tunnel: w4166 -> [w4173 w4180]
              tunnel: [w4173 w4175] -> w4162
              frame False {
              }
              frame True {
                n2168 = call-dynamic "Read AcquisitionC.vi"("error in (no error)"=w4180, "S4ACS_GUI in"=w4181) -> ("error out"=w4198:errorcluster, "Acquisition.lvclass"=w4197:refnum<class "Acquisition.lvclass">)  [unwired: 7 in, 1 out]
                n2169 = call-dynamic "Read AcquisitionA.vi"("error in (no error)"=w4180, "S4ACS_GUI in"=w4181) -> ("error out"=w4201:errorcluster, "Acquisition.lvclass"=w4202:refnum<class "Acquisition.lvclass">, "S4ACS_GUI out"=w4190:refnum<class "S4GUI.lvclass">)  [unwired: 7 in]
                n2170 = call "Read AcquisitionB.vi"("error in (no error)"=w4180, "S4ACS_GUI in"=w4181) -> ("error out"=w4199:errorcluster, "Acquisition.lvclass"=w4200:refnum<class "Acquisition.lvclass">)  [unwired: 7 in, 1 out]
                n2171 = call-dynamic "Read AcquisitionD.vi"("error in (no error)"=w4180, "S4ACS_GUI in"=w4181) -> ("error out"=w4195:errorcluster, "Acquisition.lvclass"=w4196:refnum<class "Acquisition.lvclass">)  [unwired: 7 in, 1 out]
                n2172 = call-dynamic "Read enabled.vi"("error in (no error)"=w4195, "Server in"=w4196) -> ("error out"=w4204:errorcluster, "enabled"=w4203:bool, "Server out"=w4205:refnum<class "Acquisition.lvclass">)  [unwired: 7 in]
                n2173 = call-dynamic "Read enabled.vi"("error in (no error)"=w4198, "Server in"=w4197) -> ("error out"=w4207:errorcluster, "enabled"=w4206:bool, "Server out"=w4208:refnum<class "Acquisition.lvclass">)  [unwired: 7 in]
                n2174 = call-dynamic "Read enabled.vi"("error in (no error)"=w4199, "Server in"=w4200) -> ("error out"=w4210:errorcluster, "enabled"=w4209:bool, "Server out"=w4211:refnum<class "Acquisition.lvclass">)  [unwired: 7 in]
                n2175 = call-dynamic "Read enabled.vi"("error in (no error)"=w4201, "Server in"=w4202) -> ("error out"=w4213:errorcluster, "enabled"=w4212:bool, "Server out"=w4214:refnum<class "Acquisition.lvclass">)  [unwired: 7 in]
                n2176 = case shown="True" w4209 {
                  tunnel: w4211 -> [w4294 w4298]
                  tunnel: w4210 -> [w4293 w4297]
                  tunnel: [w4294 w4296] -> w4187
                  tunnel: [w4293 w4295] -> w4186
                  frame False {
                  }
                  frame True {
                    # "Ext Start"
                    # "nome do arquivo .cfg"
                    # "seção no arquivo .cfg"
                    n2177 = call-dynamic "Read Channel.vi"("error in (no error)"=w4297, "Acquisition in"=w4298) -> ("error out"=w4302:errorcluster, "Channel.lvclass"=w4301:refnum<class "Channel.lvclass">, "Acquisition out"=w4300:refnum<class "Acquisition.lvclass">)  [unwired: 7 in]
                    n2178 = call-dynamic "Read Interface.vi"("error in (no error)"=w4302, "Channel in"=w4301) -> ("error out"=w4310:errorcluster, "Interface.lvclass"=w4311:refnum<class "Interface.lvclass">, "Channel out"=w4299:refnum<class "Channel.lvclass">)  [unwired: 7 in]
                    n2179 = call-dynamic "Get CCD_Config.vi"("error in (no error)"=w4310, "Interface in"=w4311) -> ("error out"=w4307:errorcluster, "output cluster"=w4306:T31, "Interface out"=w4312:refnum<class "Interface.lvclass">)  [unwired: 7 in]
                    n2180 = Bundle By Name(cluster=w4306, "TRIGGER_MODE"=u8 6 ("SHUTTER_MODE")) -> (w4308:T31)
                    n2181 = call-dynamic "Set CCD_Config.vi"("error in (no error)"=w4307, "input cluster"=w4308, "Interface in"=w4312) -> ("error out"=w4305:errorcluster, "Interface out"=w4313:refnum<class "Interface.lvclass">)  [unwired: 7 in]
                    n2182 = Flatten To String(anything=w4308, error in (no error)=w4305) -> (data string=w4303:string, error out=w4304:errorcluster)  [unwired: 2 in, 1 out]
                    n2183 = call "Write flatted cluster.vi"("error in (no error)"=w4304, "flatted cluster"=w4303, "Interface in"=w4313) -> ("error out"=w4315:errorcluster, "Interface out"=w4314:refnum<class "Interface.lvclass">)  [unwired: 7 in]
                    n2184 = call-dynamic "Write Interface.vi"("error in (no error)"=w4315, "Interface.lvclass"=w4314, "Channel in"=w4299) -> ("error out"=w4321:errorcluster, "Channel out"=w4322:refnum<class "Channel.lvclass">)  [unwired: 7 in]
                    n2185 = call "Write section_name.vi"("error in (no error)"=w4321, "section_name"="CCD_ACS2", "Channel in"=w4322) -> ("error out"=w4319:errorcluster, "Channel out"=w4325:refnum<class "Channel.lvclass">)  [unwired: 7 in]
                    n2186 = call-dynamic "save config.vi"("error in (no error)"=w4319, "file config"="lastsaved.cfg", "Channel in"=w4325) -> ("error out"=w4320:errorcluster, "Channel out"=w4326:refnum<class "Channel.lvclass">)  [unwired: 7 in]
                    n2187 = call-dynamic "Read State Machine.vi"("error in (no error)"=w4320, "Device in"=w4326) -> ("error out"=w4316:errorcluster, "State Machine.lvclass"=w4328:refnum<class "State Machine.lvclass">, "Device out"=w4327:refnum<class "Channel.lvclass">)  [unwired: 7 in]
                    n2188 = call-dynamic "Write State.vi"("error in (no error)"=w4316, "State"=60, "State Machine in"=w4328) -> ("error out"=w4317:errorcluster, "State Machine out"=w4329:refnum<class "State Machine.lvclass">)  [unwired: 7 in]
                    n2189 = call-dynamic "Write State Machine.vi"("error in (no error)"=w4317, "State Machine.lvclass"=w4329, "Device in"=w4327) -> ("error out"=w4331:errorcluster, "Device out"=w4330:refnum<class "Channel.lvclass">)  [unwired: 7 in]
                    n2190 = call-dynamic "Write Channel.vi"("error in (no error)"=w4331, "Channel.lvclass"=w4330, "Acquisition in"=w4300) -> ("error out"=w4295:errorcluster, "Acquisition out"=w4296:refnum<class "Acquisition.lvclass">)  [unwired: 7 in]
                  }
                }
                n2191 = case shown="True" w4212 {
                  tunnel: [w4332 w4366] -> w4188
                  tunnel: [w4333 w4365] -> w4189
                  tunnel: w4214 -> [w4333 w4335]
                  tunnel: w4213 -> [w4332 w4334]
                  frame False {
                  }
                  frame True {
                    # "nome do arquivo .cfg"
                    # "seção no arquivo .cfg"
                    # "Ext Start"
                    n2192 = call-dynamic "Read Channel.vi"("error in (no error)"=w4334, "Acquisition in"=w4335) -> ("error out"=w4367:errorcluster, "Channel.lvclass"=w4368:refnum<class "Channel.lvclass">, "Acquisition out"=w4369:refnum<class "Acquisition.lvclass">)  [unwired: 7 in]
                    n2193 = call-dynamic "Read Interface.vi"("error in (no error)"=w4367, "Channel in"=w4368) -> ("error out"=w4357:errorcluster, "Interface.lvclass"=w4356:refnum<class "Interface.lvclass">, "Channel out"=w4370:refnum<class "Channel.lvclass">)  [unwired: 7 in]
                    n2194 = call-dynamic "Get CCD_Config.vi"("error in (no error)"=w4357, "Interface in"=w4356) -> ("error out"=w4360:errorcluster, "output cluster"=w4361:T31, "Interface out"=w4355:refnum<class "Interface.lvclass">)  [unwired: 7 in]
                    n2195 = Bundle By Name(cluster=w4361, "TRIGGER_MODE"=u8 6 ("SHUTTER_MODE")) -> (w4359:T31)
                    n2196 = call-dynamic "Set CCD_Config.vi"("error in (no error)"=w4360, "input cluster"=w4359, "Interface in"=w4355) -> ("error out"=w4362:errorcluster, "Interface out"=w4354:refnum<class "Interface.lvclass">)  [unwired: 7 in]
                    n2197 = Flatten To String(anything=w4359, error in (no error)=w4362) -> (data string=w4364:string, error out=w4363:errorcluster)  [unwired: 2 in, 1 out]
                    n2198 = call "Write flatted cluster.vi"("error in (no error)"=w4363, "flatted cluster"=w4364, "Interface in"=w4354) -> ("error out"=w4352:errorcluster, "Interface out"=w4353:refnum<class "Interface.lvclass">)  [unwired: 7 in]
                    n2199 = call-dynamic "Write Interface.vi"("error in (no error)"=w4352, "Interface.lvclass"=w4353, "Channel in"=w4370) -> ("error out"=w4347:errorcluster, "Channel out"=w4346:refnum<class "Channel.lvclass">)  [unwired: 7 in]
                    n2200 = call "Write section_name.vi"("error in (no error)"=w4347, "section_name"="CCD_ACS1", "Channel in"=w4346) -> ("error out"=w4348:errorcluster, "Channel out"=w4343:refnum<class "Channel.lvclass">)  [unwired: 7 in]
                    n2201 = call-dynamic "save config.vi"("error in (no error)"=w4348, "file config"="lastsaved.cfg", "Channel in"=w4343) -> ("error out"=w4336:errorcluster, "Channel out"=w4337:refnum<class "Channel.lvclass">)  [unwired: 7 in]
                    n2202 = call-dynamic "Read State Machine.vi"("error in (no error)"=w4336, "Device in"=w4337) -> ("error out"=w4351:errorcluster, "State Machine.lvclass"=w4341:refnum<class "State Machine.lvclass">, "Device out"=w4342:refnum<class "Channel.lvclass">)  [unwired: 7 in]
                    n2203 = call-dynamic "Write State.vi"("error in (no error)"=w4351, "State"=60, "State Machine in"=w4341) -> ("error out"=w4350:errorcluster, "State Machine out"=w4340:refnum<class "State Machine.lvclass">)  [unwired: 7 in]
                    n2204 = call-dynamic "Write State Machine.vi"("error in (no error)"=w4350, "State Machine.lvclass"=w4340, "Device in"=w4342) -> ("error out"=w4338:errorcluster, "Device out"=w4339:refnum<class "Channel.lvclass">)  [unwired: 7 in]
                    n2205 = call-dynamic "Write Channel.vi"("error in (no error)"=w4338, "Channel.lvclass"=w4339, "Acquisition in"=w4369) -> ("error out"=w4366:errorcluster, "Acquisition out"=w4365:refnum<class "Acquisition.lvclass">)  [unwired: 7 in]
                  }
                }
                n2206 = case shown="True" w4206 {
                  tunnel: w4208 -> [w4255 w4259]
                  tunnel: w4207 -> [w4254 w4258]
                  tunnel: [w4255 w4257] -> w4185
                  tunnel: [w4254 w4256] -> w4184
                  frame False {
                  }
                  frame True {
                    # "Ext Start"
                    # "nome do arquivo .cfg"
                    # "seção no arquivo .cfg"
                    n2207 = call-dynamic "Read Channel.vi"("error in (no error)"=w4258, "Acquisition in"=w4259) -> ("error out"=w4263:errorcluster, "Channel.lvclass"=w4262:refnum<class "Channel.lvclass">, "Acquisition out"=w4261:refnum<class "Acquisition.lvclass">)  [unwired: 7 in]
                    n2208 = call-dynamic "Read Interface.vi"("error in (no error)"=w4263, "Channel in"=w4262) -> ("error out"=w4271:errorcluster, "Interface.lvclass"=w4272:refnum<class "Interface.lvclass">, "Channel out"=w4260:refnum<class "Channel.lvclass">)  [unwired: 7 in]
                    n2209 = call-dynamic "Get CCD_Config.vi"("error in (no error)"=w4271, "Interface in"=w4272) -> ("error out"=w4268:errorcluster, "output cluster"=w4267:T31, "Interface out"=w4273:refnum<class "Interface.lvclass">)  [unwired: 7 in]
                    n2210 = Bundle By Name(cluster=w4267, "TRIGGER_MODE"=u8 6 ("SHUTTER_MODE")) -> (w4269:T31)
                    n2211 = call-dynamic "Set CCD_Config.vi"("error in (no error)"=w4268, "input cluster"=w4269, "Interface in"=w4273) -> ("error out"=w4266:errorcluster, "Interface out"=w4274:refnum<class "Interface.lvclass">)  [unwired: 7 in]
                    n2212 = Flatten To String(anything=w4269, error in (no error)=w4266) -> (data string=w4264:string, error out=w4265:errorcluster)  [unwired: 2 in, 1 out]
                    n2213 = call "Write flatted cluster.vi"("error in (no error)"=w4265, "flatted cluster"=w4264, "Interface in"=w4274) -> ("error out"=w4276:errorcluster, "Interface out"=w4275:refnum<class "Interface.lvclass">)  [unwired: 7 in]
                    n2214 = call-dynamic "Write Interface.vi"("error in (no error)"=w4276, "Interface.lvclass"=w4275, "Channel in"=w4260) -> ("error out"=w4282:errorcluster, "Channel out"=w4283:refnum<class "Channel.lvclass">)  [unwired: 7 in]
                    n2215 = call "Write section_name.vi"("error in (no error)"=w4282, "section_name"="CCD_ACS3", "Channel in"=w4283) -> ("error out"=w4280:errorcluster, "Channel out"=w4286:refnum<class "Channel.lvclass">)  [unwired: 7 in]
                    n2216 = call-dynamic "save config.vi"("error in (no error)"=w4280, "file config"="lastsaved.cfg", "Channel in"=w4286) -> ("error out"=w4281:errorcluster, "Channel out"=w4287:refnum<class "Channel.lvclass">)  [unwired: 7 in]
                    n2217 = call-dynamic "Read State Machine.vi"("error in (no error)"=w4281, "Device in"=w4287) -> ("error out"=w4277:errorcluster, "State Machine.lvclass"=w4289:refnum<class "State Machine.lvclass">, "Device out"=w4288:refnum<class "Channel.lvclass">)  [unwired: 7 in]
                    n2218 = call-dynamic "Write State.vi"("error in (no error)"=w4277, "State"=60, "State Machine in"=w4289) -> ("error out"=w4278:errorcluster, "State Machine out"=w4290:refnum<class "State Machine.lvclass">)  [unwired: 7 in]
                    n2219 = call-dynamic "Write State Machine.vi"("error in (no error)"=w4278, "State Machine.lvclass"=w4290, "Device in"=w4288) -> ("error out"=w4292:errorcluster, "Device out"=w4291:refnum<class "Channel.lvclass">)  [unwired: 7 in]
                    n2220 = call-dynamic "Write Channel.vi"("error in (no error)"=w4292, "Channel.lvclass"=w4291, "Acquisition in"=w4261) -> ("error out"=w4256:errorcluster, "Acquisition out"=w4257:refnum<class "Acquisition.lvclass">)  [unwired: 7 in]
                  }
                }
                n2221 = case shown="True" w4203 {
                  tunnel: w4205 -> [w4216 w4220]
                  tunnel: w4204 -> [w4215 w4219]
                  tunnel: [w4216 w4218] -> w4183
                  tunnel: [w4215 w4217] -> w4182
                  frame False {
                  }
                  frame True {
                    # "Ext Start"
                    # "nome do arquivo .cfg"
                    # "seção no arquivo .cfg"
                    n2222 = call-dynamic "Read Channel.vi"("error in (no error)"=w4219, "Acquisition in"=w4220) -> ("error out"=w4250:errorcluster, "Channel.lvclass"=w4251:refnum<class "Channel.lvclass">, "Acquisition out"=w4252:refnum<class "Acquisition.lvclass">)  [unwired: 7 in]
                    n2223 = call-dynamic "Read Interface.vi"("error in (no error)"=w4250, "Channel in"=w4251) -> ("error out"=w4242:errorcluster, "Interface.lvclass"=w4241:refnum<class "Interface.lvclass">, "Channel out"=w4253:refnum<class "Channel.lvclass">)  [unwired: 7 in]
                    n2224 = call-dynamic "Get CCD_Config.vi"("error in (no error)"=w4242, "Interface in"=w4241) -> ("error out"=w4245:errorcluster, "output cluster"=w4246:T31, "Interface out"=w4240:refnum<class "Interface.lvclass">)  [unwired: 7 in]
                    n2225 = Bundle By Name(cluster=w4246, "TRIGGER_MODE"=u8 6 ("SHUTTER_MODE")) -> (w4244:T31)
                    n2226 = call-dynamic "Set CCD_Config.vi"("error in (no error)"=w4245, "input cluster"=w4244, "Interface in"=w4240) -> ("error out"=w4247:errorcluster, "Interface out"=w4239:refnum<class "Interface.lvclass">)  [unwired: 7 in]
                    n2227 = Flatten To String(anything=w4244, error in (no error)=w4247) -> (data string=w4249:string, error out=w4248:errorcluster)  [unwired: 2 in, 1 out]
                    n2228 = call "Write flatted cluster.vi"("error in (no error)"=w4248, "flatted cluster"=w4249, "Interface in"=w4239) -> ("error out"=w4237:errorcluster, "Interface out"=w4238:refnum<class "Interface.lvclass">)  [unwired: 7 in]
                    n2229 = call-dynamic "Write Interface.vi"("error in (no error)"=w4237, "Interface.lvclass"=w4238, "Channel in"=w4253) -> ("error out"=w4231:errorcluster, "Channel out"=w4230:refnum<class "Channel.lvclass">)  [unwired: 7 in]
                    n2230 = call "Write section_name.vi"("error in (no error)"=w4231, "section_name"="CCD_ACS4", "Channel in"=w4230) -> ("error out"=w4233:errorcluster, "Channel out"=w4227:refnum<class "Channel.lvclass">)  [unwired: 7 in]
